vi "torque_diagram.vi"(8 "Torque":dbl, 11 "Array in":i32[](array[numeric])) -> (3 "Array out":i32[](array[numeric]))   [LabVIEW 2014]
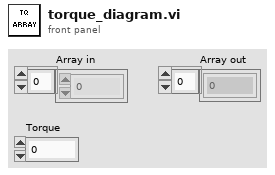
[diagram p1: front panel]
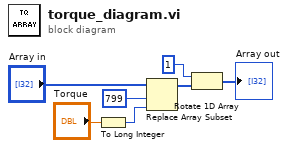
[diagram p0: block diagram]
diagram:
  n1 = To Long Integer(number="Torque") -> (32bit integer=w7:i32)
  n2 = Replace Array Subset(array="Array in", new element=w7, index=799) -> (w4:i32[])
  n3 = Rotate 1D Array(1:w4, 2:1 ("n")) -> (0:→"Array out":i32[])
